vi "Keyboard Setup.vi"(0 "String in":refnum<vi>, 1 "This VI":refnum<vi>, 2 "Hide OVR Key (T)":bool, 5 "reference in":refnum<vi>, 9 "Max Length (70)":i32=70, 11 "Password Display (F)":bool, 12 "String In":string, 13 "Message In":string) -> (4 "String Out":string, 15 "error out":errorcluster)   [LabVIEW 2015, in "Touch_keyboard.lvlib"]
doc: "This VI initializes the front panel of the Keyboard application"
uses:
  Touch_keyboard.lvlib
  Driver Commands.ctl
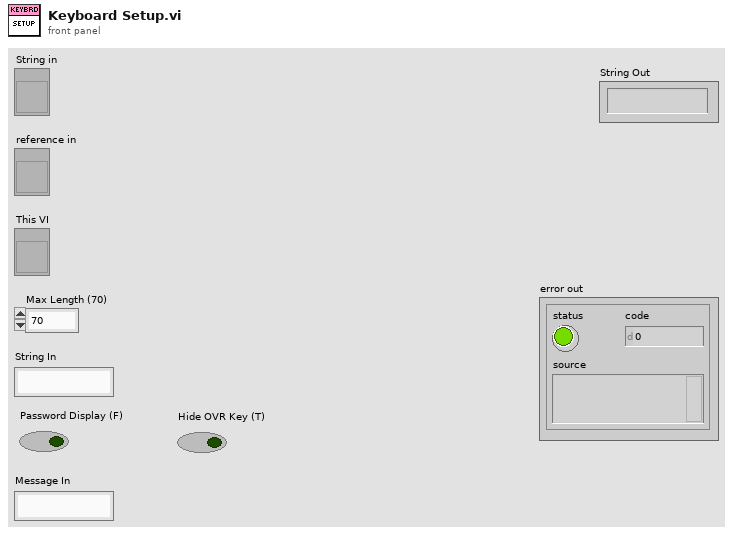
[diagram p1: front panel]
types:
  T1 = typedef "Touch_keyboard.lvlib/Driver Commands.ctl" = enum16{"No Command", "Initialize", "Add Character", "Replace Charcter", "Delete Character", "Move Left", "Move Right", "Update Edit Position"}
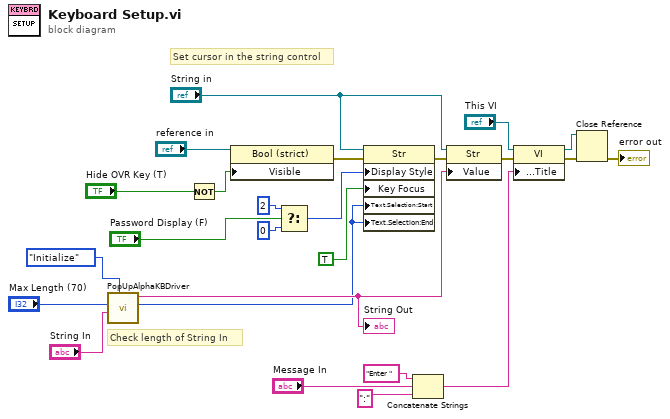
[diagram p0: block diagram]
diagram:
  # "Set cursor in the string control"
  # "Check length of String In"
  n1 = call "PopUpAlphaKBDriver.vi"("Driver Commands"=Driver_Commands."Initialize", "Initial String"="String In", "Max Length (70)"="Max Length (70)") -> ("Edit Position"=w14:i32, "String Out"=w15:string)  [unwired: 7 in]
  "String Out" <- w15
  n2 = Not(x="Hide OVR Key (T)") -> (.not. x?=w9:bool)
  n3 = property on="Property Node" class="Bool (strict)"(reference="reference in", "Visible"=w9) -> (error out=w25:errorcluster)  [unwired: 1 in, 1 out]
  n4 = Select(t=u32 2 ("Display Style"), s="Password Display (F)", f=u32 0 ("Display Style")) -> (s? t:f=w11:u32)
  n5 = property on="Property Node" class="Str"(reference="String in", error in=w25, "Display Style"=w11, "Key Focus"=TRUE, "Text.Selection:Start"=w14, "Text.Selection:End"=w14) -> (error out=w2:errorcluster)  [unwired: 1 out]
  n6 = Concatenate Strings("Enter ", "Message In", ":" ("Substring")) -> (w17:string)
  n7 = property class="Str"(reference="String in", error in=w2, "Value"=w15) -> (error out=w1:errorcluster)  [unwired: 1 out]
  n8 = property class="VI"(reference="This VI", error in=w1, "Front Panel Window:Title"=w17) -> (reference out=w19:refnum<vi>, error out=w18:errorcluster)
  n9 = Close Reference(reference=w19, error in (no error)=w18) -> (error out=→"error out":errorcluster)
